vi "Compare PrevState_State.vi"(8 "error in (no error)":errorcluster, 11 "State Machine in":refnum<class "State Machine.lvclass">) -> (0 "error out":errorcluster, 2 "prev = state ?":bool, 3 "State Machine out":refnum<class "State Machine.lvclass">)   [LabVIEW 2018, in "State Machine.lvclass"]
uses:
  State Machine.lvclass
  State Machine.lvclass/State Machine.ctl
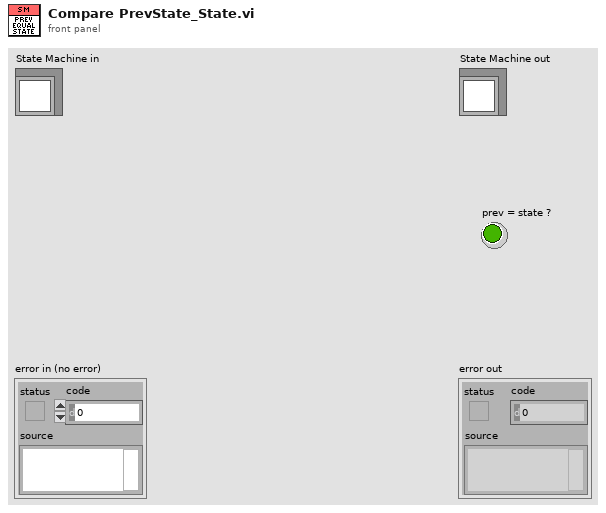
[diagram p1: front panel]
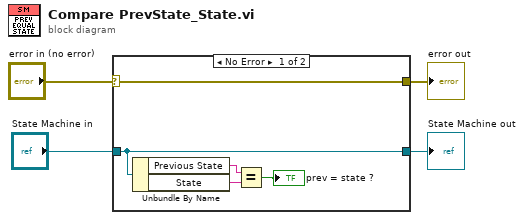
[diagram p0: block diagram]
diagram:
  n1 = case shown="No Error" "error in (no error)" {
    selector: "error in (no error)" -> [w9 w11]
    tunnel: [w9 w11] -> w3
    tunnel: [w8 w10] -> w1
    tunnel: "State Machine in" -> [w8 w10]
    frame No Error {
      n2 = Unbundle By Name(w8) -> ("Previous State"=w7:string, "State"=w6:string)
      n3 = Equal?(x=w7, y=w6) -> (x = y?=→"prev = state ?":bool)
    }
    frame Error {
    }
  }
  "error out" <- w3
  "State Machine out" <- w1
